vi "Process.vi"(8 "error in (no error)":errorcluster, 11 "RandomNumberGenerator in":refnum<class "RandomNumberGenerator.lvclass">) -> (0 "error out":errorcluster, 3 "RandomNumberGenerator out":refnum<class "RandomNumberGenerator.lvclass">)   [LabVIEW 2020, in "RandomNumberGenerator.lvlib" / "RandomNumberGenerator.lvclass"]
doc: "<b>Process</b>\nThis method is called based on the timing set in the <b>Initialize</b> or <b>Configure Session</b> methods, and is where the vast majority of the work done by your plugin will happen. Here, your plugin can read the data that was sent to the plugin (if any), perform some action(s), and optionally send data to the PEF Engine for other plugins to receive.\n\nThe Process state gets called repeatedly by the engine. You do not need to implement a while loop to continuously run in the Process state. Your process state must not call any code with an infinite timeout. \nInstead, use a defined timeout and handle/ignore the timeout error accordingly. This ensures that the system does not hang or get stuck.\n\nThere may be many instances of the same plugin running on the system. Because the state VIs in plugins run with Shared Clone reentrancy, there is no guarantee that any data stored in diagram or front panel structures (such as feedback nodes, shift registers, front panel objects, etc) are from the same instance of the plugin. Any data that needs to persist between calls to the Process VI must be persisted in the class private data of the plugin."
uses:
  RandomNumberGenerator.lvclass
  RandomNumberGenerator.lvclass/RandomNumberGenerator.ctl
  <vilib>/ADAS Record/Utilities/ADAS Utilities.lvlib
  <vilib>/ADAS Record/CustomDataTypes/Double/Process Data.ctl
  <vilib>/ADAS Record/CustomDataTypes/Double/Double.lvlib
  C:/Program Files/National Instruments/LabVIEW 2020/vi.lib/FlexLogger/SDK/PluginSDK.lvlibp/PEFClasses/SDK/Processing Element/Processing Element.lvclass
  C:/Projects/GitHub/data-record-ad/IO Plugins/RandomNumberGenerator/PE/RandomNumberGenerator.lvclass
  <vilib>/ADAS Record/CustomDataTypes/Double/Write.vi
  <vilib>/numeric/Random Number (Range) DBL.vi
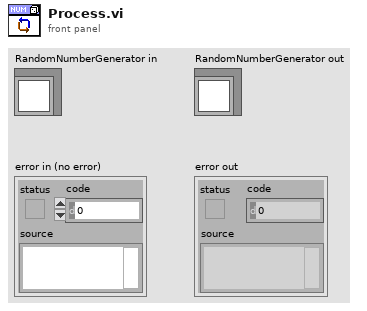
[diagram p1: front panel]
types:
  T1 = typedef "Double.lvlib/Process Data.ctl" = cluster{"Time Stamp":timestamp, "Double (DBL)":dbl}
  T2 = typedef "RandomNumberGenerator.lvlib/RandomNumberGenerator.lvclass/Configuration.ctl" = cluster{"Lower Bound":dbl, "Upper Bound":dbl, "# Elements":i32, "Update Rate (ms)":i32}
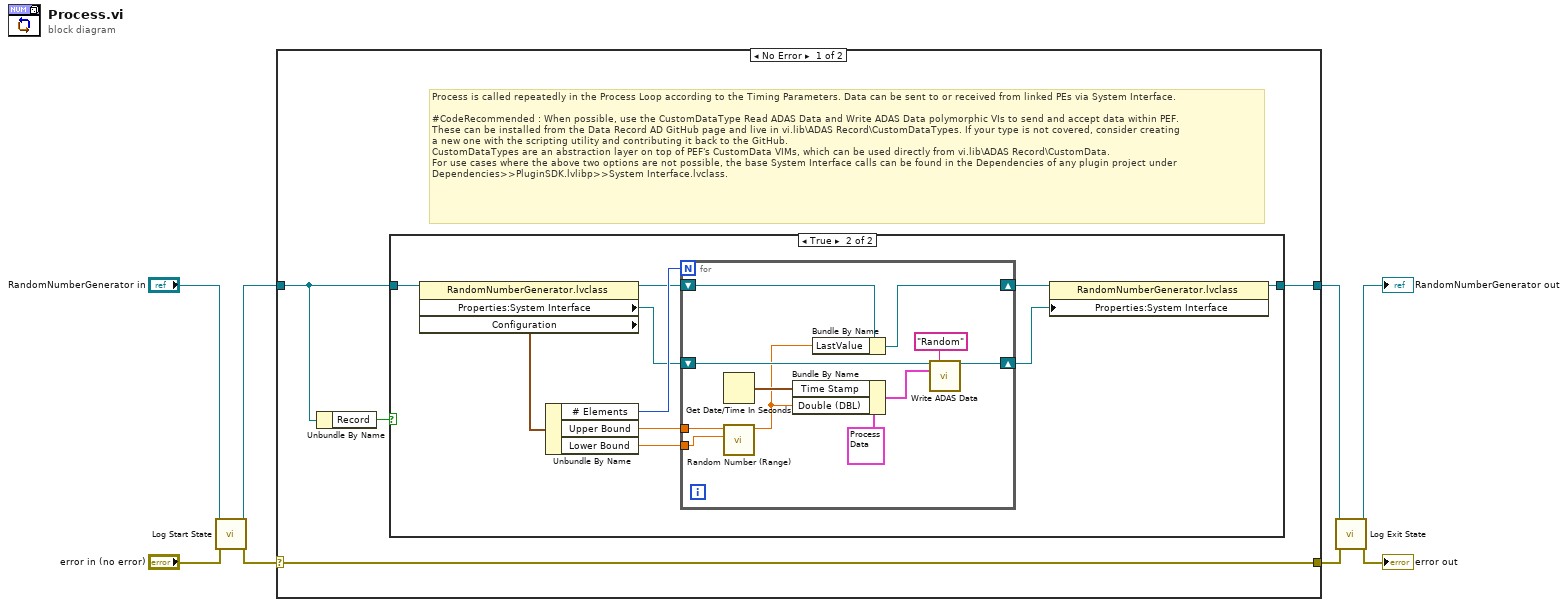
[diagram p0: block diagram]
diagram:
  n1 = call <vilib>:"Log Start State.vi"("error in (no error)"="error in (no error)", "PluginSDK.lvlibp:Processing Element.lvclass"="RandomNumberGenerator in") -> ("error out"=w7:errorcluster, "PluginSDK.lvlibp:Processing Element.lvclass"=w5:refnum<class "RandomNumberGenerator.lvclass">)  [unwired: 8 in]
  n2 = case shown="No Error" w7 {
    selector: w7 -> [w12 w35]
    tunnel: [w11 w36] -> w2
    tunnel: w5 -> [w10 w36]
    tunnel: [w12 w35] -> w4
    frame No Error {
      # "Process is called repeatedly in the Process Loop according to the Timing Parameters. Data can be sent to or received from linked PEs via System Interface.\n\n#CodeRecommended : When possible, use the CustomDataType Read ADAS Data and Write ADAS Data polymorphic VIs to send and accept data within PEF.\nThese can be installed from the Data Record AD GitHub page and live in vi.lib\\ADAS Record\\CustomDataTypes. If your type is not covered, consider creating\na new one with the scripting utility and contributing it back to the GitHub.\nCustomDataTypes are an abstraction layer on top of PEF's CustomData VIMs, which can be used directly from vi.lib\\ADAS Record\\CustomData.\nFor use cases where the above two options are not possible, the base System Interface calls can be found in the Dependencies of any plugin project under\nDependencies>>PluginSDK.lvlibp>>System Interface.lvclass."
      n3 = Unbundle By Name(w10) -> ("Record"=w9:bool)
      n4 = case shown="True" w9 {
        tunnel: [w13 w17] -> w11
        tunnel: w10 -> [w13 w16]
        frame False {
        }
        frame True {
          n5 = property on="Property Node" class="RandomNumberGenerator.lvclass"(reference=w16) -> (reference out=w15:refnum<class "RandomNumberGenerator.lvclass">, "Properties:System Interface"=w19:refnum<class "System Interface.lvclass">, "Configuration"=w23:T2)  [unwired: 1 in, 1 out]
          n6 = Unbundle By Name(w23) -> ("# Elements"=w22:i32, "Upper Bound"=w21:dbl, "Lower Bound"=w20:dbl)
          n7 = for {
            N: w22 -> [_]
            tunnel: w21 -> [w34]
            tunnel: w20 -> [w33]
            shift-right: [w31] -> w18
            shift-left: w19 -> [w32]
            shift-right: [w25] -> w14
            shift-left: w15 -> [w26]
            n8 = Get Date/Time In Seconds() -> (seconds since 1Jan1904=w27:timestamp)
            n9 = call-poly <vilib>:"Random Number (Range).vi"("lower bound (0)"=w33, "upper bound (100)"=w34) -> ("number"=w24:dbl)  [unwired: 9 in]
            n10 = Bundle By Name(cluster=T1 {"Time Stamp"=timestamp(0 s since 1904-01-01), "Double (DBL)"=0.0} ("Process Data"), "Time Stamp"=w27, "Double (DBL)"=w24) -> (w28:T1)
            n11 = Bundle By Name(cluster=w26, "LastValue"=w24) -> (w25:refnum<class "RandomNumberGenerator.lvclass">)
            n12 = call-poly <vilib>:"Write ADAS Data.vi"("System Interface"=w32, "Terminal"="Random", "Process Data"=w28) -> ("System Interface out"=w31:refnum<class "System Interface.lvclass">)  [unwired: 11 in, 1 out]
          }
          n13 = property on="Property Node" class="RandomNumberGenerator.lvclass"(reference=w14, "Properties:System Interface"=w18) -> (reference out=w17:refnum<class "RandomNumberGenerator.lvclass">)  [unwired: 1 in, 1 out]
        }
      }
    }
    frame Error {
    }
  }
  n14 = call <vilib>:"Log Exit State.vi"("error in (no error)"=w4, "PluginSDK.lvlibp:Processing Element.lvclass"=w2) -> ("error out"=→"error out":errorcluster, "PluginSDK.lvlibp:Processing Element.lvclass"=→"RandomNumberGenerator out":refnum<class "RandomNumberGenerator.lvclass">)  [unwired: 8 in]
